vi "4-2 난수발생.vi"() -> ()   [LabVIEW 2014]
panel:
  out "웨이브폼 차트":dbl(graph)
  in  "경로":path=path "C:/Users/LVEDU09/Desktop/a.bmp"
  in  "메뉴바/도구바":bool
  in  "정지":bool
  in  "난수발생":bool
  in  "가운데로":bool
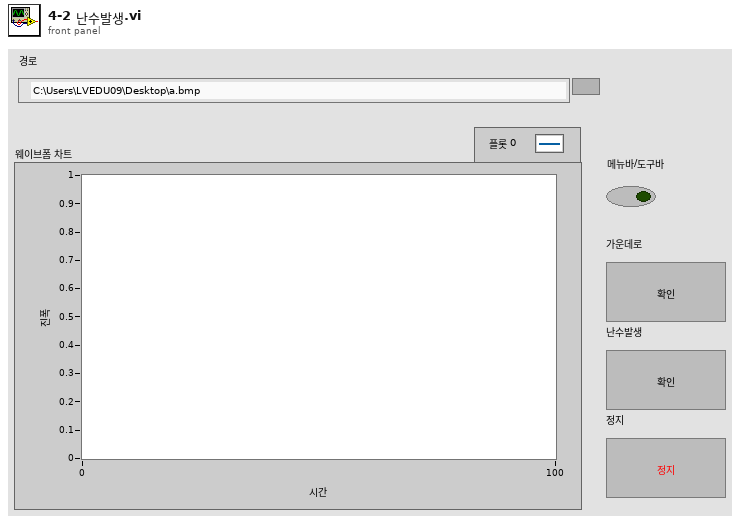
[diagram p1: front panel]
types:
  T1 = enum16{"Always On", "Always Off", "Off While Running"}
  T2 = enum32{"invalid app kind", "Development System", "Run Time System", "Student Edition", "Embedded LabVIEW", "Evaluation", "Custom"}
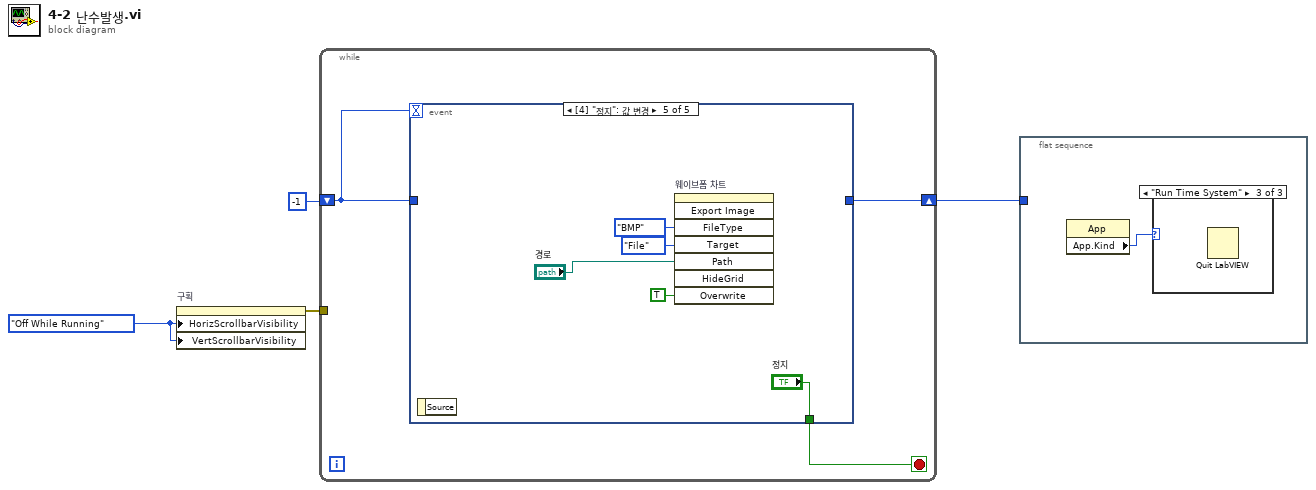
[diagram p0: block diagram]
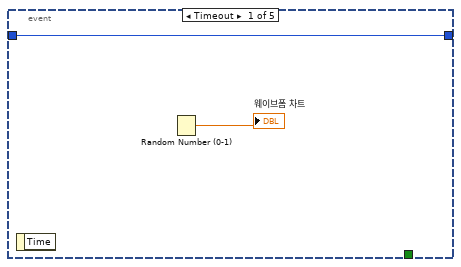
[diagram p4: hidden frame]
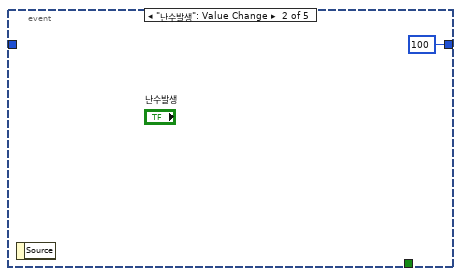
[diagram p5: hidden frame]
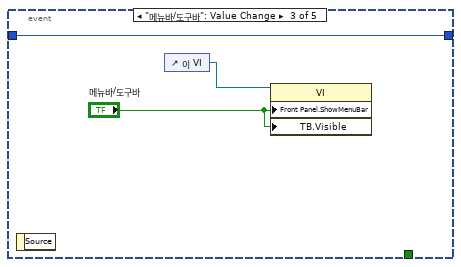
[diagram p6: hidden frame]
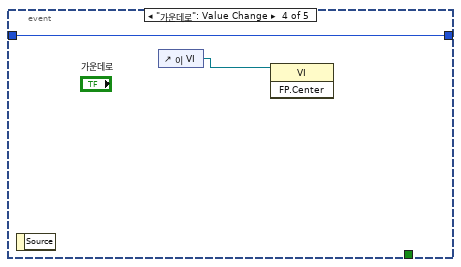
[diagram p7: hidden frame]
diagram:
  w3 = T1."Off While Running" ("수평 스크롤 막대 보이기")
  n1 = property on="구획" class="Pane"("HorizScrollbarVisibility"=w3, "VertScrollbarVisibility"=w3) -> (error out=w2:errorcluster)  [unwired: 2 in, 1 out]
  n2 = while {
    shift-right: [w6] -> w1
    shift-left: -1 -> [w7]
    tunnel: w2 -> [_]
    stop <- w5 stop-if-true
    n3 = event shown="[4] \"정지\": 값 변경" {
      selector: _ -> [_ _ _ _ _]
      dyn-events: _ -> [_ _ _ _ _]
      timeout: w7 -> [_ _ _ _ _]
      tunnel: w7 -> [w9 _ w11 w14 _]
      tunnel: [w9 100 w11 w14 _] -> w6
      tunnel: [_ _ _ _ "정지"] -> w5
      event Timeout {
        n4 = event-data() -> ()  [unwired: 1 in, 1 out]
        n5 = Random Number (0-1)() -> (number: 0 to 1=→"웨이브폼 차트":dbl)
      }
      event "난수발생": Value Change {
        n6 = event-data() -> ()  [unwired: 1 in, 1 out]
      }
      event "메뉴바/도구바": Value Change {
        n7 = event-data() -> ()  [unwired: 1 in, 1 out]
        n8 = control-ref of="이 VI"() -> (w13:refnum<vi>)
        n9 = property class="VI"(reference=w13, "Front Panel.ShowMenuBar"="메뉴바/도구바", "TB.Visible"="메뉴바/도구바") -> ()  [unwired: 1 in, 2 out]
      }
      event "가운데로": Value Change {
        n10 = event-data() -> ()  [unwired: 1 in, 1 out]
        n11 = control-ref of="이 VI"() -> (w15:refnum<vi>)
        n12 = invoke class="VI" method="FP.Center"(reference=w15) -> ()  [unwired: 2 in, 3 out]
      }
      event "정지": Value Change {
        n13 = event-data() -> ()  [unwired: 1 in, 1 out]
        n14 = invoke on="웨이브폼 차트" class="WFChart (엄격한)" method="Export Image"("FileType"=enum32{"BMP", "EPS", "EMF", "PICT"}."BMP" ("파일 타입"), "Target"=enum32{"File", "Clipboard"}."File" ("타겟"), "Path"="경로", "Overwrite"=TRUE ("항상 덮어쓰기")) -> ()  [unwired: 4 in, 8 out]
      }
    }
  }
  n15 = flat-sequence {
    tunnel: w1 -> [_]
    frame #0 {
      n16 = property class="App"() -> ("App.Kind"=w21:T2)  [unwired: 2 in, 2 out]
      n17 = case shown="\"Run Time System\"" w21 {
        frame "invalid app kind", Default {
        }
        frame "Development System" {
        }
        frame "Run Time System" {
          n18 = Quit LabVIEW() -> ()  [unwired: 1 in]
        }
      }
    }
  }
